vi "DataSocket Write Connections Manager.vi"(10 "URL":string, 11 "Action":enum16{"Get", "Close", "Close All"}(ring)) -> (0 "error out":errorcluster, 3 "connection id":refnum<k13>)   [LabVIEW 2024]
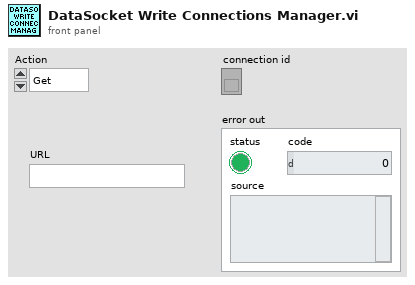
[diagram p1: front panel]
types:
  T1 = enum16{"Read", "Write", "ReadWrite", "BufferedRead", "BufferedReadWrite"}
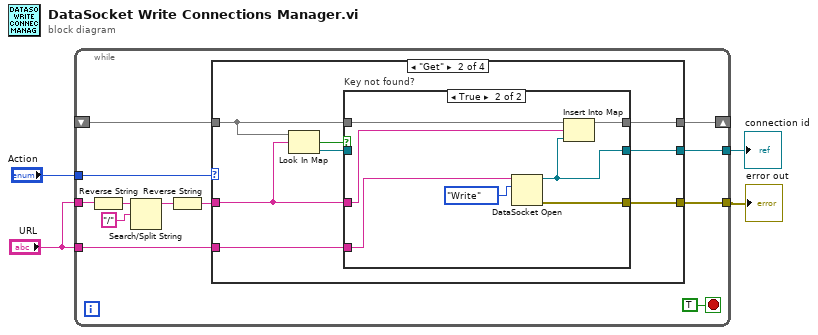
[diagram p0: block diagram]
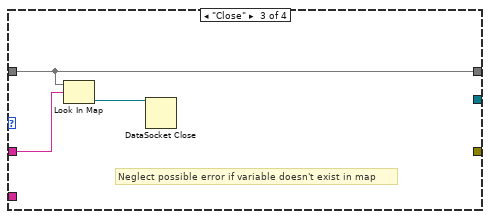
[diagram p4: hidden frame]
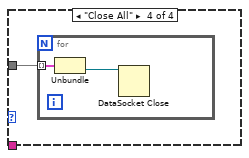
[diagram p5: hidden frame]
diagram:
  n1 = while {
    shift-right: [w14] -> _
    shift-left: _ -> [w13]
    tunnel: "URL" -> [w8]
    tunnel: [w12] -> w3
    tunnel: "Action" -> [w15]
    tunnel: "URL" -> [w6]
    tunnel: [w5] -> w1
    stop <- TRUE stop-if-true
    n2 = Reverse String(1:w8) -> (0:w11:string)
    n3 = Search/Split String(string=w11, search string/char (-)="/") -> (substring before match=w9:string)  [unwired: 1 in, 2 out]
    n4 = Reverse String(1:w9) -> (0:w7:string)
    n5 = case shown="\"Get\"" w15 {
      tunnel: [_ w22 w34 _] -> w14
      tunnel: w13 -> [_ w23 w34 w37]
      tunnel: w7 -> [_ w21 w36 _]
      tunnel: [_ w19 _ _] -> w12
      tunnel: w6 -> [_ w18 _ _]
      tunnel: [_ w17 _ _] -> w5
      frame Default {
      }
      frame "Get" {
        n6 = Look In Map(map=w23, key=w21) -> (key not found?=w24:bool, value=w20:refnum<k13>)  [unwired: 1 in]
        n7 = case "Key not found?" shown="True" w24 {
          tunnel: w23 -> [w25 w33]
          tunnel: [w25 w32] -> w22
          tunnel: w21 -> [_ w29]
          tunnel: w20 -> [w26 _]
          tunnel: [w26 w31] -> w19
          tunnel: w18 -> [_ w28]
          tunnel: [_ w27] -> w17
          frame False {
          }
          frame True {
            n8 = DataSocket Open(10:T1."Write" ("mode"), 11:w28) -> (0:w27:errorcluster, 3:w31:refnum<k13>)  [unwired: 2 in]
            n9 = Insert Into Map(map in=w33, key=w29, value=w31) -> (map out=w32:map{string, refnum<k13>})  [unwired: 2 out]
          }
        }
      }
      frame "Close" {
        # "Neglect possible error if variable doesn't exist in map"
        n10 = Look In Map(map=w34, key=w36) -> (value=w35:refnum<k13>)  [unwired: 1 in, 1 out]
        n11 = DataSocket Close(11:w35) -> ()  [unwired: 2 in, 2 out]
      }
      frame "Close All" {
        n12 = for {
          tunnel: w37 -> [w39] mode=indexing
          n13 = Unbundle(w39) -> ("connection id"=w38:refnum<k13>)  [unwired: 1 out]
          n14 = DataSocket Close(11:w38) -> ()  [unwired: 2 in, 2 out]
        }
      }
    }
  }
  "connection id" <- w3
  "error out" <- w1
